vi "organize files.vi"() -> ()   [LabVIEW 2016]
panel:
  out "Number of files choosen":i32
  in  "format string":string="%06d.itx"
  out "Index chosen":dbl[](array[numeric])
  in  "Interested Loop":i32
  in  "Loop number":i32
  in  "Offset for each loop":dbl[](array[numeric])
  in  "Numbers of each loop":dbl[](array[numeric])
  out "error out 2":errorcluster
  in  "fileName part1":string
  in  "error in":errorcluster
  in  "Move to":path
  in  "Move from":path
  # "Notice: (Downward: Inner loop to Outer)"
  # "Loop from outter to inner: ...-4-3-2-1-0"
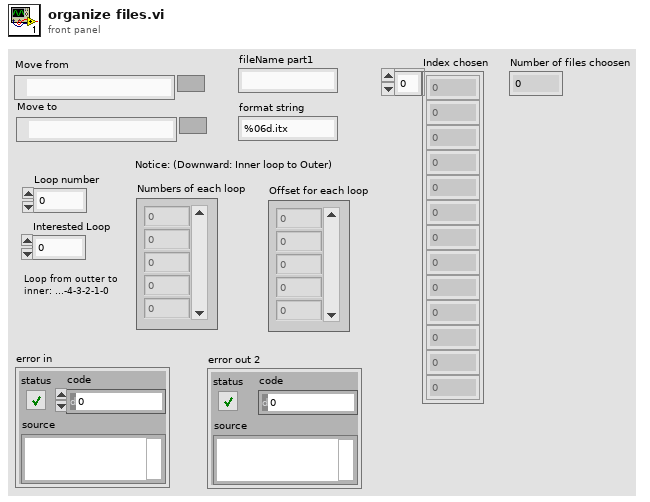
[diagram p1: front panel]
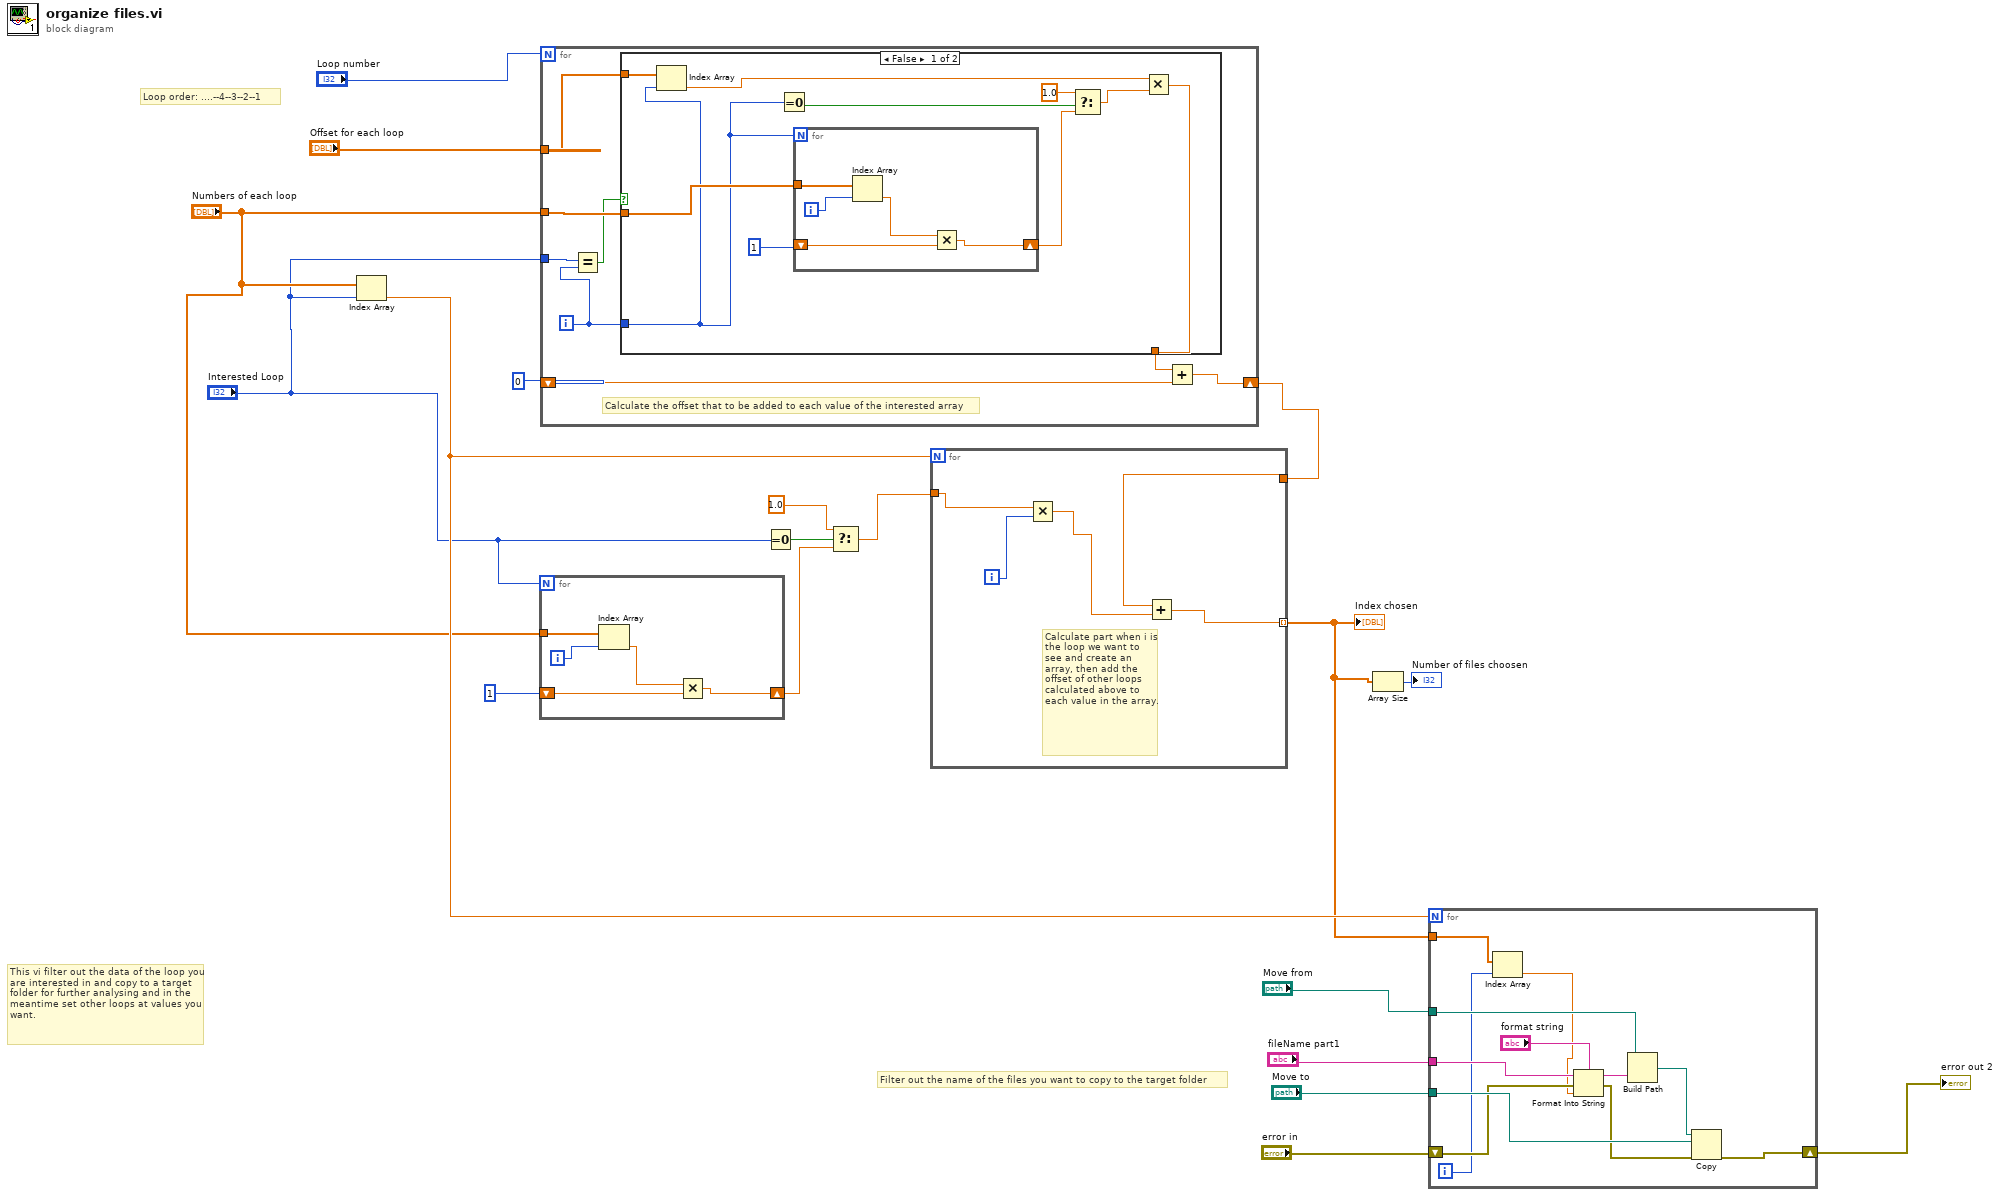
[diagram p0: block diagram]
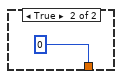
[diagram p2: hidden frame]
diagram:
  # "Filter out the name of the files you want to copy to the target folder"
  # "Loop order: ....--4--3--2--1"
  # "This vi filter out the data of the loop you are interested in and copy to a target folder for further analysing and in the meantime set other loops at values you want."
  n1 = Index Array(array="Numbers of each loop", index="Interested Loop") -> (element=w16:dbl)
  n2 = for {
    N: "Interested Loop" -> [_]
    tunnel: "Numbers of each loop" -> [w22]
    shift-right: [w20] -> w12
    shift-left: 1 -> [w24]
    i -> [w23]
    n3 = Index Array(array=w22, index=w23) -> (element=w21:dbl)
    n4 = Multiply(x=w21, y=w24) -> (x*y=w20:dbl)
  }
  n5 = for {
    N: "Loop number" -> [_]
    tunnel: "Numbers of each loop" -> [w28]
    tunnel: "Offset for each loop" -> [w32]
    shift-right: [w30] -> w15
    shift-left: 0 -> [w31]
    tunnel: "Interested Loop" -> [w27]
    i -> [w26]
    # "Calculate the offset that to be added to each value of the interested array"
    n6 = Equal?(x=w27, y=w26) -> (x = y?=w25:bool)
    n7 = case shown="False" w25 {
      tunnel: w32 -> [w42 _]
      tunnel: [w35 0] -> w29
      tunnel: w28 -> [w34 _]
      tunnel: w26 -> [w33 _]
      frame False {
        n8 = Index Array(array=w42, index=w33) -> (element=w38:dbl)
        n9 = Equal To 0?(x=w33) -> (x = 0?=w40:bool)
        n10 = for {
          N: w33 -> [_]
          tunnel: w34 -> [w45]
          shift-right: [w43] -> w39
          shift-left: 1 -> [w47]
          i -> [w46]
          n11 = Index Array(array=w45, index=w46) -> (element=w44:dbl)
          n12 = Multiply(x=w44, y=w47) -> (x*y=w43:dbl)
        }
        n13 = Select(t=1.0, s=w40, f=w39) -> (s? t:f=w37:dbl)
        n14 = Multiply(x=w38, y=w37) -> (x*y=w35:dbl)
      }
      frame True {
      }
    }
    n15 = Add(x=w29, y=w31) -> (x+y=w30:dbl)
  }
  n16 = Equal To 0?(x="Interested Loop") -> (x = 0?=w8:bool)
  n17 = Select(t=1.0, s=w8, f=w12) -> (s? t:f=w11:dbl)
  n18 = for {
    N: w16 -> [_]
    tunnel: w15 -> [w52]
    tunnel: [w51] -> w2 mode=indexing
    tunnel: w11 -> [w49]
    i -> [w50]
    # "Calculate part when i is the loop we want to see and create an array, then add the offset of other loops calculated above to each value in the array."
    n19 = Multiply(x=w49, y=w50) -> (x*y=w53:dbl)
    n20 = Add(x=w52, y=w53) -> (x+y=w51:dbl)
  }
  "Index chosen" <- w2
  n21 = Array Size(array=w2) -> (size(s)=→"Number of files choosen":i32)
  n22 = for {
    N: w16 -> [_]
    tunnel: "Move to" -> [w65]
    tunnel: "Move from" -> [w64]
    tunnel: "fileName part1" -> [w62]
    shift-right: [w57] -> w6
    shift-left: "error in" -> [w59]
    tunnel: w2 -> [w56]
    i -> [w55]
    n23 = Index Array(array=w56, index=w55) -> (element=w54:dbl)
    n24 = Format Into String(format string="format string", initial string=w62, error in=w59, w54) -> (resulting string=w61:string, error out=w58:errorcluster)
    n25 = Build Path(base path=w64, name or relative path=w61) -> (appended path=w60:path)
    n26 = Copy(8:w58, 10:w65, 11:w60) -> (0:w57:errorcluster)  [unwired: 2 in, 2 out]
  }
  "error out 2" <- w6
